vi "RWA_Insert Anything into String.vi"(5 "Read/Write Options":T1={"TS Fmt"="%04Y%02m%02d %02H%02M%S%25u", "Int Fmt"="%d", "Delimiter"=""}, 7 "Format String (%#_13g)":string="%#_13g", 8 "Error":errorcluster, 9 "Section Name (Name Of \"Anything\")":string, 10 "Anything":variant, 11 "File String":string) -> (0 "Error Out":errorcluster, 1 "Write Warnings Out":string, 2 "Section Replaced? Out":bool, 3 "File String Out":string)   [LabVIEW 2023]
doc: "This VI is designed to write any data type to an INI file in human readable form. It will overwrite any data in the specified section of the INI file but leave other sections unchanged.\n\nAuthored by Robert C. Mortensen\nsupport@mooregoodideas.com\nwww.mooregoodideas.com\n\nCopyright (c) 2010, Moore Good Ideas, Inc.\n\nAll rights reserved.\n\nRedistribution and use in source and binary forms, with or without modification, are permitted provided that the following conditions are met:\n\n * Redistributions of source code must retain the above copyright notice, this list of conditions and the following disclaimer.\n * Redistributions in binary form must reproduce the above copyright notice, this list of conditions and the following disclaimer in the documentation and/or other materials provided with the distribution.\n * Neither the name of Moore Good Ideas, Inc. nor the names of its contributors may be used to endorse or promote products derived from this software without specific prior written permission.\n\nTHIS SOFTWARE IS PROVIDED BY THE COPYRIGHT HOLDERS AND CONTRIBUTORS \"AS IS\" AND ANY EXPRESS OR IMPLIED WARRANTIES, INCLUDING, BUT NOT LIMITED TO, THE IMPLIED WARRANTIES OF MERCHANTABILITY AND FITNESS FOR A PARTICULAR PURPOSE ARE DISCLAIMED. IN NO EVENT SHALL THE COPYRIGHT OWNER OR CONTRIBUTORS BE LIABLE FOR ANY DIRECT, INDIRECT, INCIDENTAL, SPECIAL, EXEMPLARY, OR CONSEQUENTIAL DAMAGES (INCLUDING, BUT NOT LIMITED TO, PROCUREMENT OF SUBSTITUTE GOODS OR SERVICES; LOSS OF USE, DATA, OR PROFITS; OR BUSINESS INTERRUPTION) HOWEVER CAUSED AND ON ANY THEORY OF LIABILITY, WHETHER IN CONTRACT, STRICT LIABILITY, OR TORT (INCLUDING NEGLIGENCE OR OTHERWISE) ARISING IN ANY WAY OUT OF THE USE OF THIS SOFTWARE, EVEN IF ADVISED OF THE POSSIBILITY OF SUCH DAMAGE."
uses:
  MGI RWA Options Cluster.ctl
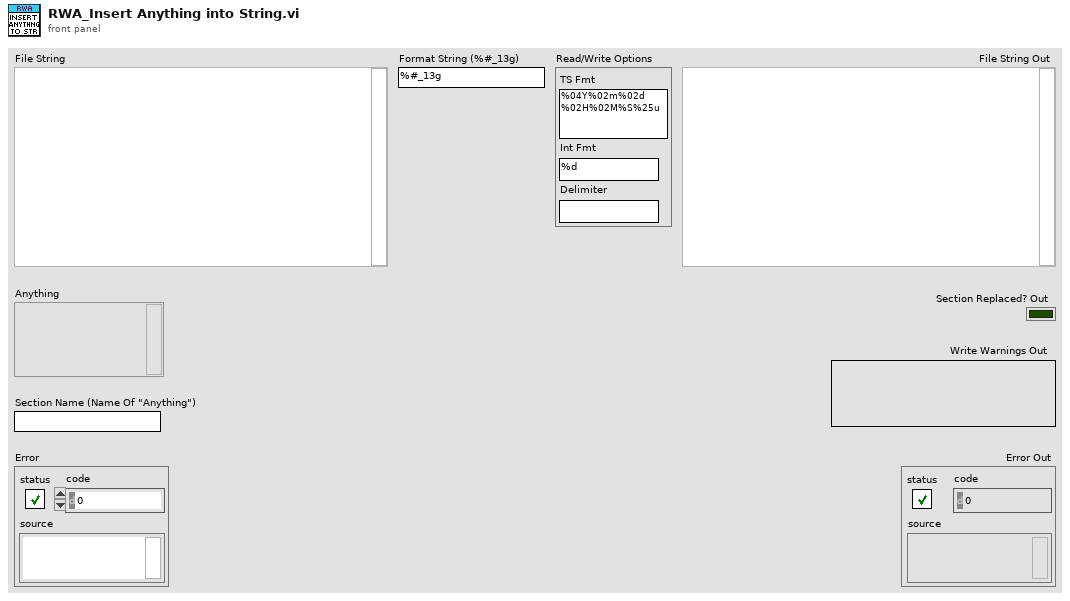
[diagram p1: front panel]
types:
  T1 = typedef "MGI RWA Options Cluster.ctl" = cluster{"TS Fmt":string, "Int Fmt":string, "Delimiter":string}
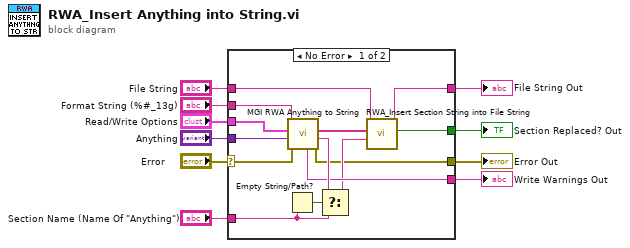
[diagram p0: block diagram]
diagram:
  n1 = case shown="No Error" "Error" {
    selector: "Error" -> [w17 w26]
    tunnel: "Anything" -> [w24 _]
    tunnel: [w11 w26] -> w9
    tunnel: "File String" -> [w12 w25]
    tunnel: "Format String (%#_13g)" -> [w23 _]
    tunnel: "Section Name (Name Of \"Anything\")" -> [w20 _]
    tunnel: "Read/Write Options" -> [w19 _]
    tunnel: [w14 _] -> w4
    tunnel: [w18 _] -> w3
    tunnel: [w13 w25] -> w1
    frame No Error {
      n2 = Empty String/Path?(string/path=w20) -> (empty?=w22:bool)
      n3 = call "MGI RWA Anything to String.vi"("Error In"=w17, "Anything"=w24, "Read/Write Options"=w19, "Format String (%#_13g)"=w23) -> ("Error Out"=w11:errorcluster, "Section"=w21:string, "Strings[]"=w16:string[], "Warnings"=w18:string)  [unwired: 4 in]
      n4 = Select(t=w21, s=w22, f=w20) -> (s? t:f=w15:string)
      n5 = call "RWA_Insert Section String into File String.vi"("Section Name"=w15, "Strings[]"=w16, "File String"=w12) -> ("Section Replaced Out"=w14:bool, "File String Out"=w13:string)  [unwired: 7 in]
    }
    frame Error {
    }
  }
  "Error Out" <- w9
  "Section Replaced? Out" <- w4
  "Write Warnings Out" <- w3
  "File String Out" <- w1
